vi "String array to limits cluster.vi"(0 "Channel Values in":string[](array[string])) -> (1 "Limits out":T1=[{"Max"=15.0, "Min"=-15.0}, {"Max"=250.0, "Min"=0.0}, {"Max"=15.0, "Min"=-15.0}] {"Min" format="%#.1f"; "Max" format="%#.1f"}, 2 "Channel Values out":string[](array[string]))   [LabVIEW 2014]
uses:
  Box_size.ctl
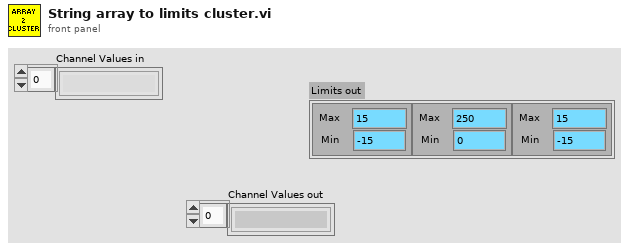
[diagram p1: front panel]
types:
  T1 = typedef "Box_size.ctl" = cluster{"Max":sgl, "Min":sgl}[]
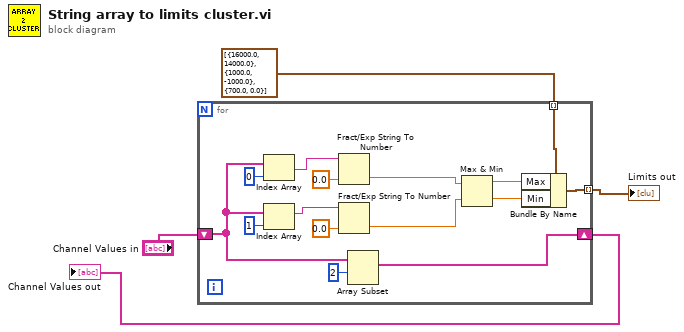
[diagram p0: block diagram]
diagram:
  n1 = for {
    shift-right: [w17] -> w4
    shift-left: "Channel Values in" -> [w16]
    tunnel: T1 [{"Max"=16000.0, "Min"=14000.0}, {"Max"=1000.0, "Min"=-1000.0}, {"Max"=700.0, "Min"=0.0}] ("Entire Space") -> [w12] mode=indexing
    tunnel: [w11] -> w1 mode=indexing
    n2 = Index Array(array=w16, index=0 ("Index")) -> (element=w14:string)
    n3 = Index Array(array=w16, index=1 ("Index")) -> (element=w13:string)
    n4 = Fract/Exp String To Number(string=w14, default (0 dbl)=sgl 0.0 ("default (0 DBL)")) -> (number=w10:sgl)  [unwired: 3 out]
    n5 = Fract/Exp String To Number(string=w13, default (0 dbl)=sgl 0.0 ("default (0 DBL)")) -> (number=w9:sgl)  [unwired: 3 out]
    n6 = Array Subset(array=w16, index=2 ("Array Index")) -> (w17:string[])  [unwired: 1 in]
    n7 = Max & Min(x=w10, y=w9) -> (max(x,y)=w8:sgl, min(x,y)=w7:sgl)
    n8 = Bundle By Name(cluster=w12, "Max"=w8, "Min"=w7) -> (w11:cluster{"Max":sgl, "Min":sgl})
  }
  "Channel Values out" <- w4
  "Limits out" <- w1
